vi "TempF_simulator.vi"() -> (0 "Farhenheit":dbl(slide) scale=0.0..100.0)   [LabVIEW 2017]
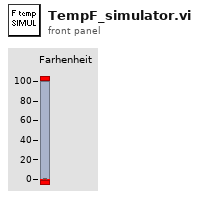
[diagram p1: front panel]
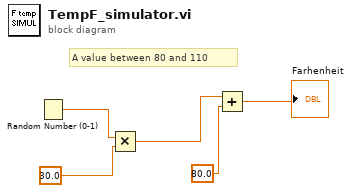
[diagram p0: block diagram]
diagram:
  # "A value between 80 and 110"
  n1 = Random Number (0-1)() -> (number: 0 to 1=w5:dbl)
  n2 = Multiply(x=w5, y=30.0) -> (x*y=w4:dbl)
  n3 = Add(x=w4, y=80.0) -> (x+y=→"Farhenheit":dbl)
